vi "Bidirectional Streaming RouteGuide Test.vi"() -> ()   [LabVIEW 2019, in "route_guide_client.lvlib"]
uses:
  route_guide_client.lvlib
  RPC Messages/routeguide_RouteNote.ctl
  RPC Messages/routeguide_Point.ctl
panel:
  in  "stop":bool
  out "Response Data":T1
  in  "Request Data":T1
  in  "Server Address":string="localhost:50051"
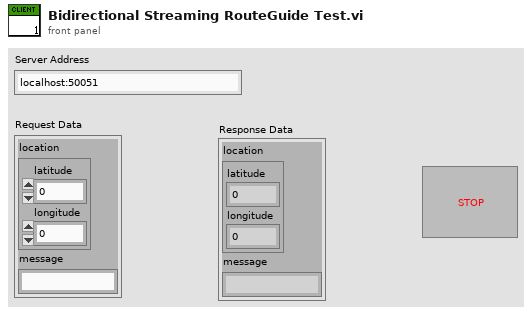
[diagram p1: front panel]
types:
  T1 = typedef "route_guide_client.lvlib/routeguide_RouteNote.ctl" = cluster{"location":T2, "message":string}
  T2 = typedef "route_guide_client.lvlib/routeguide_Point.ctl" = cluster{"latitude":i32, "longitude":i32}
  T3 = typedef "gprc-lvsupport-release.lvlib/grpcId.ctl" = u64
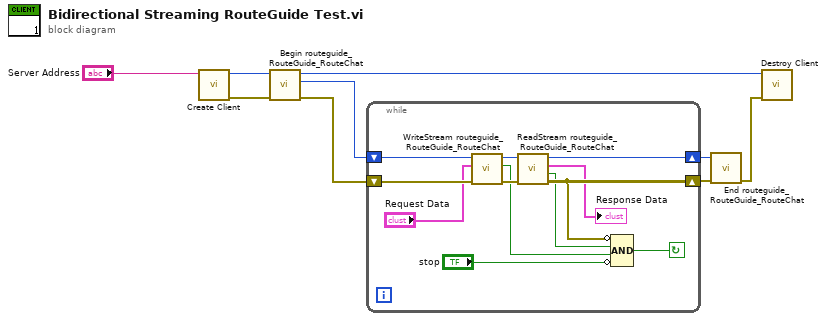
[diagram p0: block diagram]
diagram:
  n1 = call "Create Client.vi"("address"="Server Address") -> ("error out"=w7:errorcluster, "gRPC ID Out"=w8:T3)  [unwired: 9 in]
  n2 = call "Begin routeguide_RouteGuide_RouteChat.vi"("error in"=w7, "gRPC ID"=w8) -> ("error out"=w3:errorcluster, "Call Id Out"=w6:T3, "gRPC ID out"=w1:T3)  [unwired: 7 in]
  n3 = while {
    shift-right: [w18] -> w5
    shift-left: w6 -> [w21]
    shift-right: [w12] -> w4
    shift-left: w3 -> [w17]
    stop <- w11 continue-if-true
    n4 = call "WriteStream routeguide_RouteGuide_RouteChat.vi"("error in"=w17, "Request Data"="Request Data", "Call ID in"=w21) -> ("error out"=w19:errorcluster, "Success"=w13:bool, "Call ID"=w20:T3)  [unwired: 6 in]
    n5 = call "ReadStream routeguide_RouteGuide_RouteChat.vi"("error in"=w19, "Call ID in"=w20) -> ("error out"=w12:errorcluster, "Success"=w14:bool, "Response Data"=→"Response Data":T1, "Call ID"=w18:T3)  [unwired: 6 in]
    n6 = Compound Arithmetic op=AND(invert w12, w14, w13, invert "stop") -> (w11:bool)
  }
  n7 = call "End routeguide_RouteGuide_RouteChat.vi"("error in"=w4, "Call ID in"=w5) -> ("error out"=w2:errorcluster)  [unwired: 8 in, 1 out]
  n8 = call "Destroy Client.vi"("error in"=w2, "gRPC ID"=w1) -> ()  [unwired: 9 in, 1 out]
